vi "Fc_2update_graph.vi"(9 "Cluster in":T1, 10 "Local Mode":enum32{"Resume", "Hold"}(ring), 11 "WaveformGraph in":refnum<vi>) -> (2 "Cluster out":T1, 3 "Update Waveform Graph":bool)   [LabVIEW 2022 SP3]
doc: "This function updates the waveform graph."
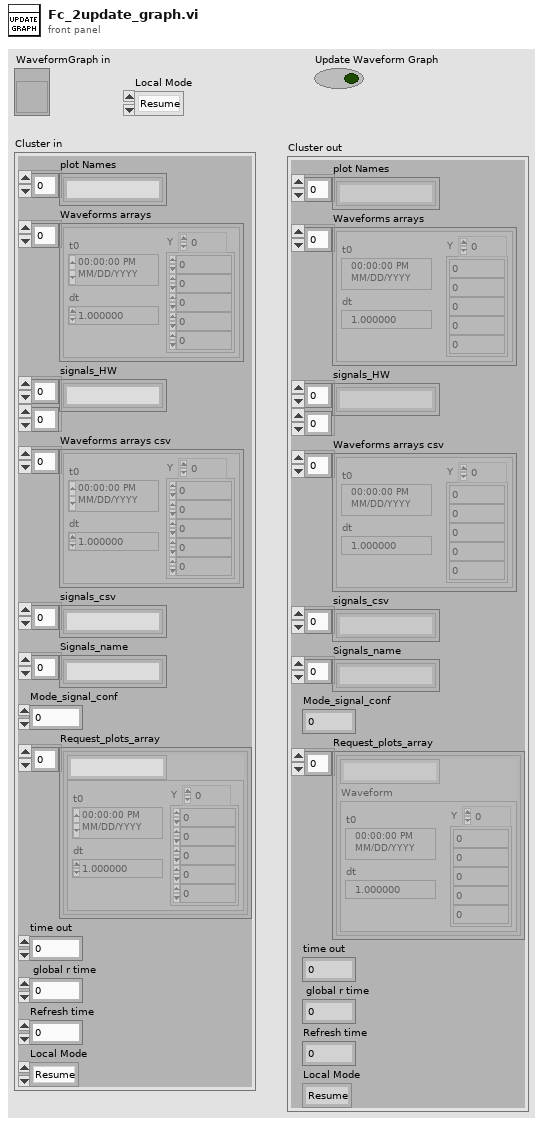
[diagram p1: front panel]
types:
  T1 = cluster{"plot Names":string[], "Waveforms arrays":waveform(dbl)[], "signals_HW":string[][], "Waveforms arrays csv":waveform(dbl)[], "signals_csv":string[], "Signals_name":string[], "Mode_signal_conf":u8, "Request_plots_array":cluster{string, "Waveform":waveform(dbl)}[], "time out":i32, " global r time":u32, "Refresh time":u32, "Local Mode":enum32{"Resume", "Hold"}}
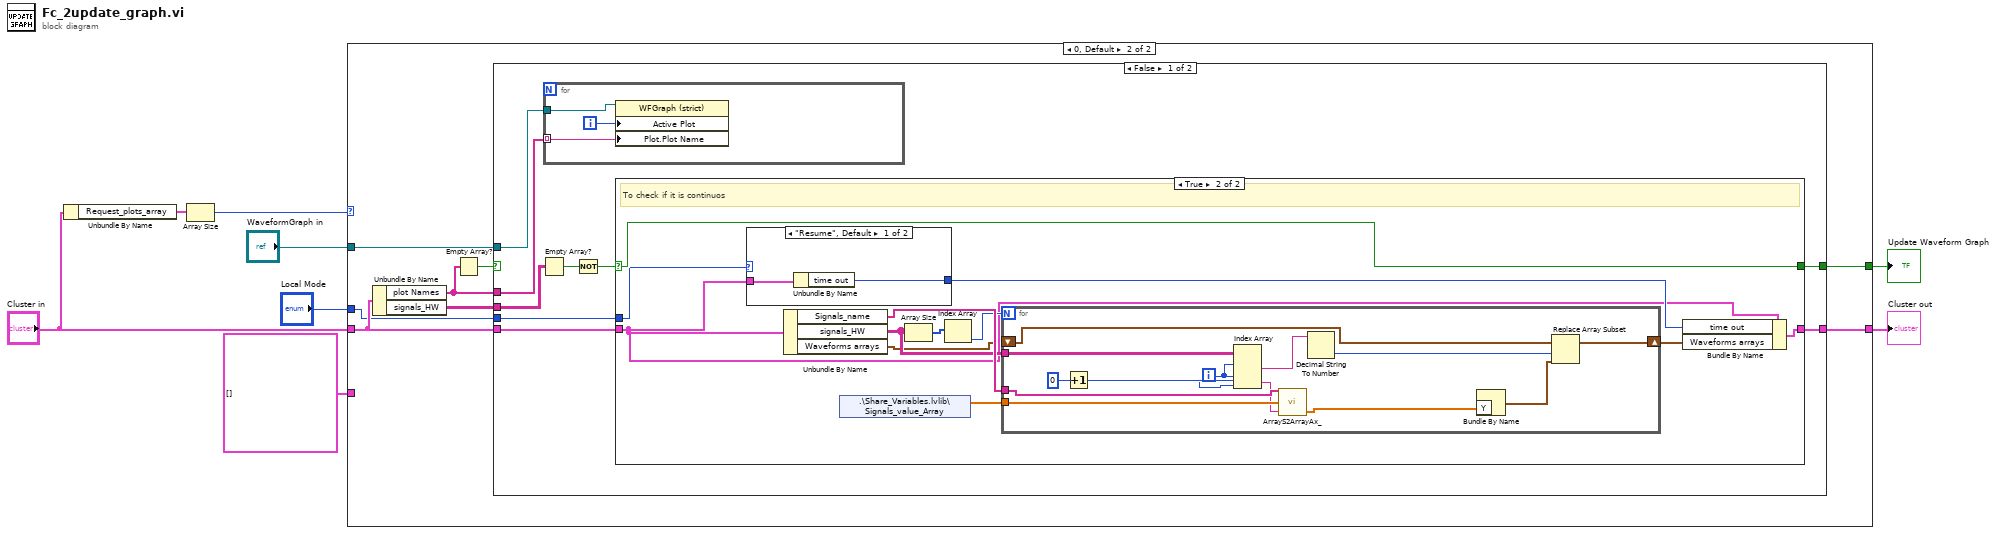
[diagram p0: block diagram]
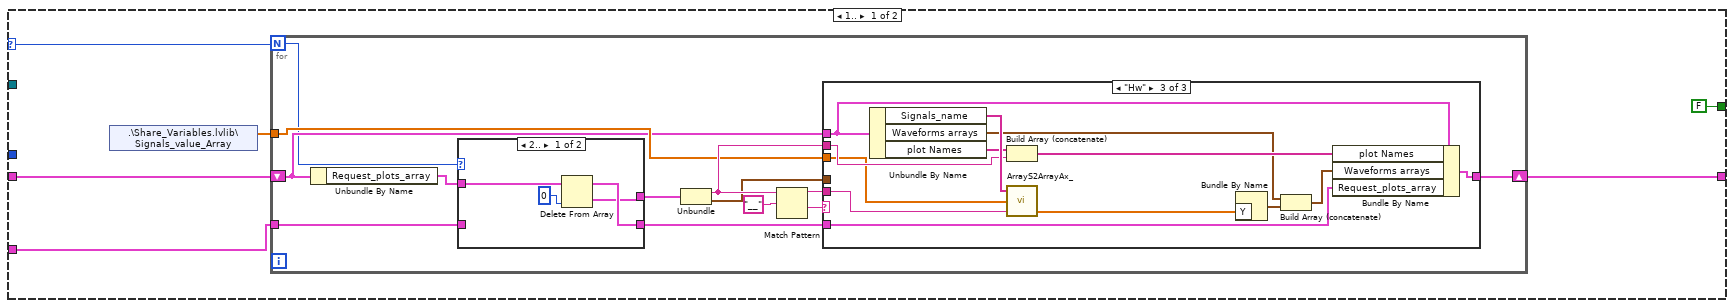
[diagram p2: hidden frame]
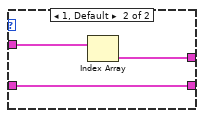
[diagram p3: hidden frame]
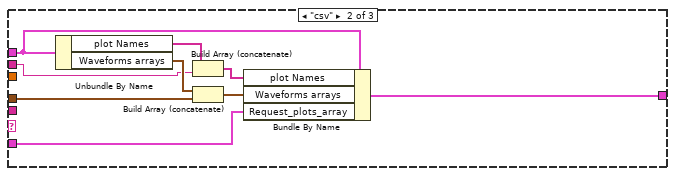
[diagram p5: hidden frame]
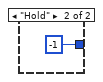
[diagram p7: hidden frame]
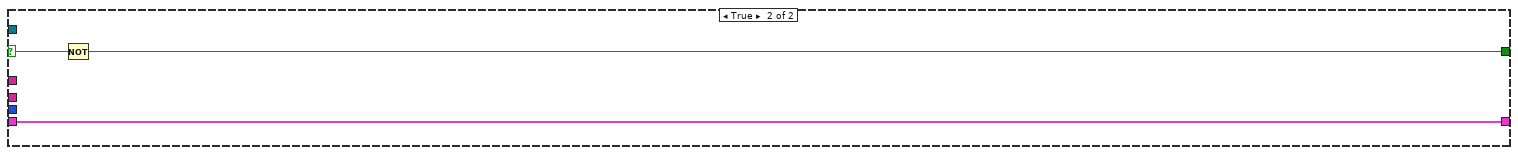
[diagram p8: hidden frame]
diagram:
  n1 = Unbundle By Name("Cluster in") -> ("Request_plots_array"=w5:cluster{string, "Waveform":waveform(dbl)}[])
  n2 = Array Size(array=w5) -> (size(s)=w6:i32)
  n3 = case shown="0, Default" w6 {
    selector: w6 -> [w10 _]
    tunnel: "Cluster in" -> [w13 w63]
    tunnel: [w14 w62] -> w7
    tunnel: [FALSE w60] -> w8
    tunnel: "WaveformGraph in" -> [_ w59]
    tunnel: "Local Mode" -> [_ w58]
    tunnel: cluster{string, "Waveform":waveform(dbl)}[] [] ("Request_plots_array") -> [w9 _]
    frame 1.. {
      n4 = shared-variable ".\\Share_Variables.lvlib\\Signals_value_Array"() -> (w11:dbl[])  [unwired: 1 in, 1 out]
      n5 = for {
        N: w10 -> [w15]
        tunnel: w11 -> [w21]
        shift-right: [w24] -> w14
        shift-left: w13 -> [w20]
        tunnel: w9 -> [w17]
        n6 = Unbundle By Name(w20) -> ("Request_plots_array"=w16:cluster{string, "Waveform":waveform(dbl)}[])
        n7 = case shown="2.." w15 {
          tunnel: w16 -> [w30 w34]
          tunnel: [w29 w32] -> w19
          tunnel: [w28 w33] -> w18
          tunnel: w17 -> [_ w32]
          frame 2.. {
            n8 = Delete From Array(array=w30, index=0) -> (deleted portion=w28:cluster{string, "Waveform":waveform(dbl)}, array with subset deleted=w29:cluster{string, "Waveform":waveform(dbl)}[])  [unwired: 1 in]
          }
          frame 1, Default {
            n9 = Index Array(array=w34) -> (element=w33:cluster{string, "Waveform":waveform(dbl)})  [unwired: 1 in]
          }
        }
        n10 = Unbundle(w18) -> (w23:string, "Waveform"=w22:waveform(dbl))
        n11 = Match Pattern(string=w23, regular expression="__") -> (before substring=w25:string, after substring=w26:string)  [unwired: 1 in, 2 out]
        n12 = case shown="\"Hw\"" w26 {
          tunnel: w20 -> [w35 w44 w54]
          tunnel: w25 -> [_ _ w56]
          tunnel: w22 -> [_ w41 _]
          tunnel: w23 -> [_ w39 w53]
          tunnel: [w35 w37 w49] -> w24
          tunnel: w19 -> [_ w36 w47]
          tunnel: w21 -> [_ _ w45]
          frame "False", Default {
          }
          frame "csv" {
            n13 = Unbundle By Name(w44) -> ("plot Names"=w43:string[], "Waveforms arrays"=w42:waveform(dbl)[])
            n14 = Build Array (concatenate)(w43, w39) -> (w38:string[])
            n15 = Build Array (concatenate)(w42, w41) -> (w40:waveform(dbl)[])
            n16 = Bundle By Name(cluster=w44, "plot Names"=w38, "Waveforms arrays"=w40, "Request_plots_array"=w36) -> (w37:T1)
          }
          frame "Hw" {
            n17 = Unbundle By Name(w54) -> ("Signals_name"=w57:string[], "Waveforms arrays"=w46:waveform(dbl)[], "plot Names"=w48:string[])
            n18 = Build Array (concatenate)(w48, w53) -> (w52:string[])
            n19 = call "ArrayS2ArrayAx_.vi"("Signal_input"=w56, "Signals_value_Array"=w45, "Signals_name"=w57) -> ("Subarray 1x_out"=w55:sgl[])  [unwired: 2 out]
            n20 = Bundle By Name("Y"=w55) -> (w51:waveform(sgl))  [unwired: 1 in]
            n21 = Build Array (concatenate)(w46, w51) -> (w50:waveform(dbl)[])
            n22 = Bundle By Name(cluster=w54, "plot Names"=w52, "Waveforms arrays"=w50, "Request_plots_array"=w47) -> (w49:T1)
          }
        }
      }
    }
    frame 0, Default {
      n23 = Unbundle By Name(w63) -> ("plot Names"=w65:string[], "signals_HW"=w61:string[][])
      n24 = Empty Array?(array=w65) -> (empty?=w64:bool)
      n25 = case shown="False" w64 {
        selector: w64 -> [_ w109]
        tunnel: w65 -> [w74 _]
        tunnel: w61 -> [w72 _]
        tunnel: w63 -> [w73 w110]
        tunnel: [w69 w110] -> w62
        tunnel: [w68 w108] -> w60
        tunnel: w59 -> [w67 _]
        tunnel: w58 -> [w66 _]
        frame False {
          n26 = Empty Array?(array=w72) -> (empty?=w71:bool)
          n27 = for {
            tunnel: w74 -> [w106] mode=indexing
            tunnel: w67 -> [w105]
            i -> [w107]
            n28 = property on="Property Node" class="WFGraph (strict)"(reference=w105, "Active Plot"=w107, "Plot.Plot Name"=w106) -> ()  [unwired: 1 in, 2 out]
          }
          n29 = Not(x=w71) -> (.not. x?=w70:bool)
          n30 = case shown="True" w70 {
            selector: w70 -> [w75 w79]
            tunnel: w73 -> [w76 w80]
            tunnel: [w76 w83] -> w69
            tunnel: [w75 w79] -> w68
            tunnel: w66 -> [_ w78]
            frame False {
            }
            frame True {
              # "To check if it is continuos"
              n31 = case shown="\"Resume\", Default" w78 {
                tunnel: [w89 -1 ("time out")] -> w82
                tunnel: w80 -> [w90 _]
                frame "Resume", Default {
                  n32 = Unbundle By Name(w90) -> ("time out"=w89:i32)
                }
                frame "Hold" {
                }
              }
              n33 = Unbundle By Name(w80) -> ("Signals_name"=w87:string[], "signals_HW"=w86:string[][], "Waveforms arrays"=w77:waveform(dbl)[])
              n34 = shared-variable ".\\Share_Variables.lvlib\\Signals_value_Array"() -> (w88:dbl[])  [unwired: 1 in, 1 out]
              n35 = Array Size(array=w86) -> (size(s)=w85:i32[])
              n36 = Index Array(array=w85) -> (element=w84:i32)  [unwired: 1 in]
              n37 = for {
                N: w84 -> [_]
                tunnel: w86 -> [w102]
                tunnel: w88 -> [w104]
                tunnel: w87 -> [w103]
                shift-right: [w96] -> w81
                shift-left: w77 -> [w98]
                i -> [w95]
                w93 = 0 ("disabled index (row)")
                n38 = Increment(x=w93) -> (x+1=w92:i32)
                n39 = Index Array(array=w102, index (row) #1=w95, index (col) #1=w93, index (row) #2=w95, index (col) #2=w92) -> (element #1=w101:string, element #2=w94:string)
                n40 = call "ArrayS2ArrayAx_.vi"("Signal_input"=w94, "Signals_value_Array"=w104, "Signals_name"=w103) -> ("Subarray 1x_out"=w100:sgl[])  [unwired: 2 out]
                n41 = Decimal String To Number(string=w101) -> (number=w97:i32)  [unwired: 2 in, 1 out]
                n42 = Bundle By Name("Y"=w100) -> (w99:waveform(sgl))  [unwired: 1 in]
                n43 = Replace Array Subset(array=w98, new element=w99, index=w97) -> (w96:waveform(dbl)[])
              }
              n44 = Bundle By Name(cluster=w80, "time out"=w82, "Waveforms arrays"=w81) -> (w83:T1)
            }
          }
        }
        frame True {
          n45 = Not(x=w109) -> (.not. x?=w108:bool)
        }
      }
    }
  }
  "Update Waveform Graph" <- w8
  "Cluster out" <- w7
